vi "CAHistogram.vi"(2 "Peak File?":bool, 3 "index":i32, 4 "all rows":sgl[][](array[numeric]) format="%0.3f", 5 "Data":dbl[][](array[numeric])) -> (0 "Histogram":T1(graph), 1 "number":i32)   [LabVIEW 2022 SP3]
uses:
  <vilib>/Utility/file.llb/Read Delimited Spreadsheet (DBL).vi
  <vilib>/Analysis/baseanly.llb/Unimode.vi
  <vilib>/Analysis/NI_AALBase.lvlib
panel:
  in  "Load new peak file":bool
  out "mode":dbl format="%0.2f"
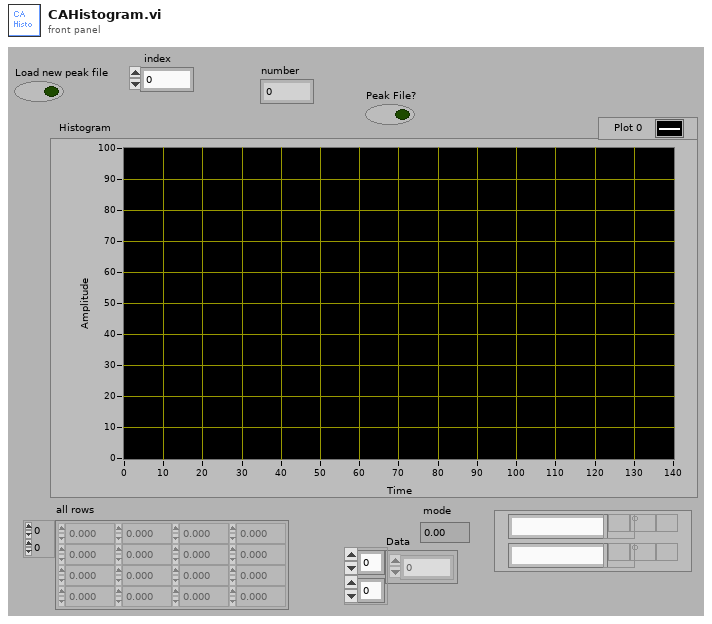
[diagram p1: front panel]
types:
  T1 = cluster{"X Values":dbl[], "Histogram: h(x)":i32[]}
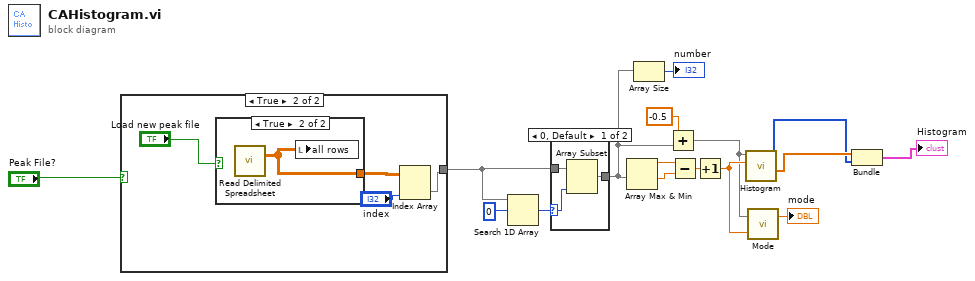
[diagram p0: block diagram]
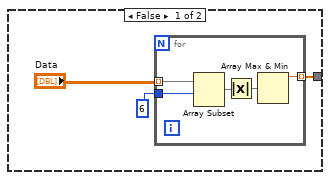
[diagram p2: hidden frame]
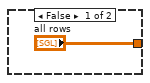
[diagram p3: hidden frame]
diagram:
  n1 = case shown="True" "Peak File?" {
    tunnel: [w18 w25] -> w1
    frame False {
      n2 = for {
        tunnel: "Data" -> [w24] mode=indexing
        tunnel: 6 -> [w23]
        tunnel: [w22] -> w18 mode=indexing
        n3 = Array Subset(array=w24, index=w23) -> (w21:dbl[])  [unwired: 1 in]
        n4 = Absolute Value(x=w21) -> (abs(x)=w20:dbl[])
        n5 = Array Max & Min(array=w20) -> (max value=w22:dbl)  [unwired: 3 out]
      }
    }
    frame True {
      n6 = case shown="True" "Load new peak file" {
        tunnel: ["all rows" w30] -> w27
        frame False {
        }
        frame True {
          n7 = call-poly <vilib>:"Read Delimited Spreadsheet.vi"() -> ("all rows"=w30:dbl[][])  [unwired: 10 in, 5 out]
          n8 = local write "all rows"(w30) -> ()
        }
      }
      n9 = Index Array(array=w27, index (col)="index") -> (element=w25:dbl[])  [unwired: 1 in]
    }
  }
  n10 = Search 1D Array(1D array=w1, element=0) -> (index of element=w7:i32)  [unwired: 1 out]
  n11 = case shown="0, Default" w7 {
    selector: w7 -> [w31 _]
    tunnel: w1 -> [w33 w34]
    tunnel: [w32 w34] -> w4
    frame 0, Default {
      n12 = Array Subset(array=w33, length=w31) -> (w32:dbl[])  [unwired: 1 in]
    }
    frame -1 {
    }
  }
  n13 = Array Max & Min(array=w4) -> (max value=w12:dbl, min value=w11:dbl)  [unwired: 2 out]
  n14 = Array Size(array=w4) -> (size(s)=→"number":i32)
  n15 = Add(x=-0.5, y=w4) -> (x+y=w6:dbl[])
  n16 = Subtract(x=w12, y=w11) -> (x-y=w10:dbl)
  n17 = Increment(x=w10) -> (x+1=w9:dbl)
  n18 = call <vilib>:"Histogram.vi"("intervals"=w9, "X"=w6) -> ("X Values"=w15:dbl[], "Histogram: h(x)"=w14:i32[])  [unwired: 8 out]
  n19 = call-poly <vilib>:"Mode.vi"("intervals"=w9, "X"=w6) -> ("mode"=→"mode":dbl)  [unwired: 1 out]
  n20 = Bundle("X Values"=w15, "Histogram: h(x)"=w14) -> (→"Histogram":T1)  [unwired: 1 out]
